vi "globalTearDown.vi"(8 "error in":errorcluster, 11 "Deployment in":refnum<class "Deployment.lvclass">) -> (0 "error out":errorcluster, 3 "Deployment out":refnum<class "Deployment.lvclass">)   [LabVIEW 2020, in "Deployment.lvclass"]
uses:
  Deployment.lvclass
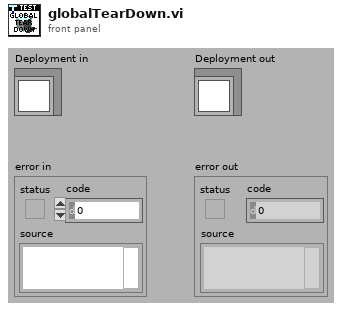
[diagram p1: front panel]
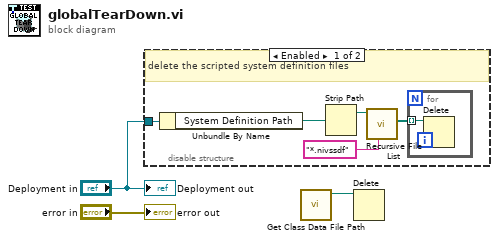
[diagram p0: block diagram]
diagram:
  n1 = disable-structure shown="Enabled" {
    disable-tunnel: "Deployment in" -> [w8 _]
    frame Enabled {
      # "delete the scripted system definition files"
      n2 = Unbundle By Name(w8) -> ("System Definition Path"=w5:path)
      n3 = Strip Path(path=w5) -> (stripped path=w4:path)  [unwired: 1 out]
      n4 = call <vilib>:"Recursive File List.vi"("pattern"="*.nivssdf", "Folder Path"=w4) -> ("All Files in Dir"=w6:path[])  [unwired: 5 in, 4 out]
      n5 = for {
        tunnel: w6 -> [w9] mode=indexing
        n6 = Delete(path (use dialog)=w9) -> ()  [unwired: 4 in, 3 out]
      }
    }
    frame Disabled {
    }
  }
  n7 = call "Get Class Data File Path.vi"() -> ("Class Data File Path"=w1:path)  [unwired: 11 in]
  n8 = Delete(path (use dialog)=w1) -> ()  [unwired: 4 in, 3 out]
  "error out" <- "error in"
  "Deployment out" <- "Deployment in"
